vi "multi_eval_template.vi"(8 "Error In":errorcluster, 10 "Data":variant, 11 "Elements":T1[](array[typedef])) -> (0 "Error Out":errorcluster, 3 "Elements out":T1[](array[typedef]))   [LabVIEW 2016]
uses:
  TypeDefs/element.ctl
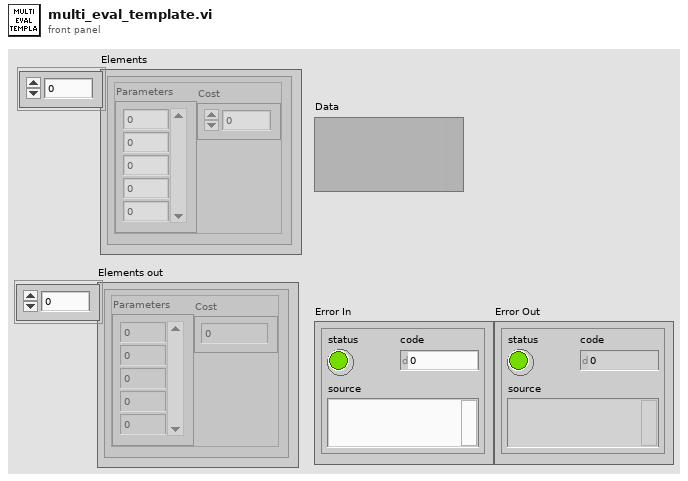
[diagram p1: front panel]
types:
  T1 = typedef "element.ctl" = cluster{"Parameters":dbl[], "Cost":dbl}
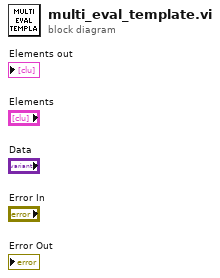
[diagram p0: block diagram]
diagram:
